vi "Create Instrument Addon From Configuration File.vi"(7 "Target in":refnum<k24>, 8 "error in (no error)":errorcluster, 11 "CD Config Path (.dat)":path) -> (0 "error out":errorcluster, 2 "Message Channels refnums":T2(array[cluster]) {"Message Group Ref" format="%.0x"; "Message Channels Refs" format="%.0x"}, 3 "Instrument Addon Refnum":T1=18446744073709551615 format="%.0x", 5 "Target out":refnum<k24>)   [LabVIEW 2018, in "Instrument Addon Scripting API.lvlib"]
uses:
  Instrument Addon Scripting API.lvlib
  <vilib>/NI Veristand/Custom Device API/Custom Device Item Ref.ctl
  NationalInstruments.VeriStand.SystemDefinitionAPI
  Addon/Addon Shared/SubVIs/Constants.vi
  <vilib>/NI Veristand/Custom Device Tools/Custom Device Utility Library/NI VeriStand - Search for All Items by GUID.vi
  <vilib>/NI Veristand/Custom Device Tools/Custom Device Utility Library/Custom Device Utility Library.lvlib
  Addon/Addon Shared/Instrument Addon Shared.lvlib
  <vilib>/NI/NI VeriStand Custom Device Import and Export Tool/ImportExport.lvlib
  <vilib>/NI Veristand/Custom Device API/Custom Device API.lvlib
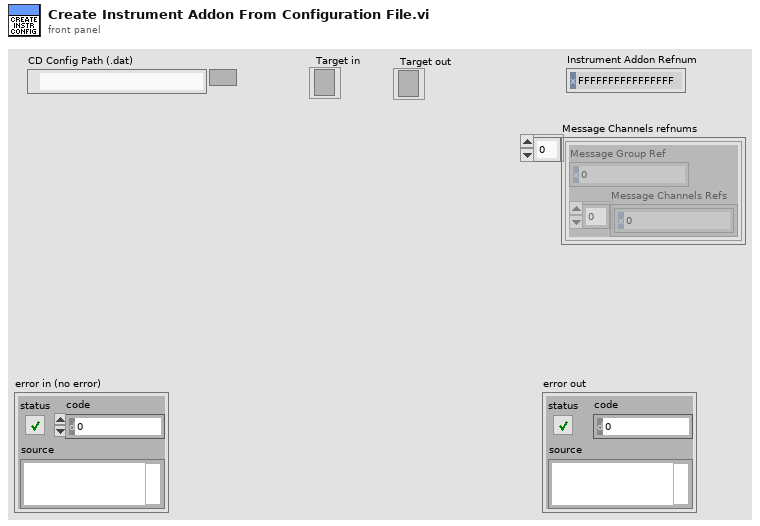
[diagram p1: front panel]
types:
  T1 = typedef "Custom Device API.lvlib/Custom Device Item Ref.ctl" = u64
  T2 = cluster{"Message Group Ref":T1, "Message Channels Refs":T1[]}[]
  T3 = cluster{"Message Group Ref":T1, "Message Channels Refs":T1[]}
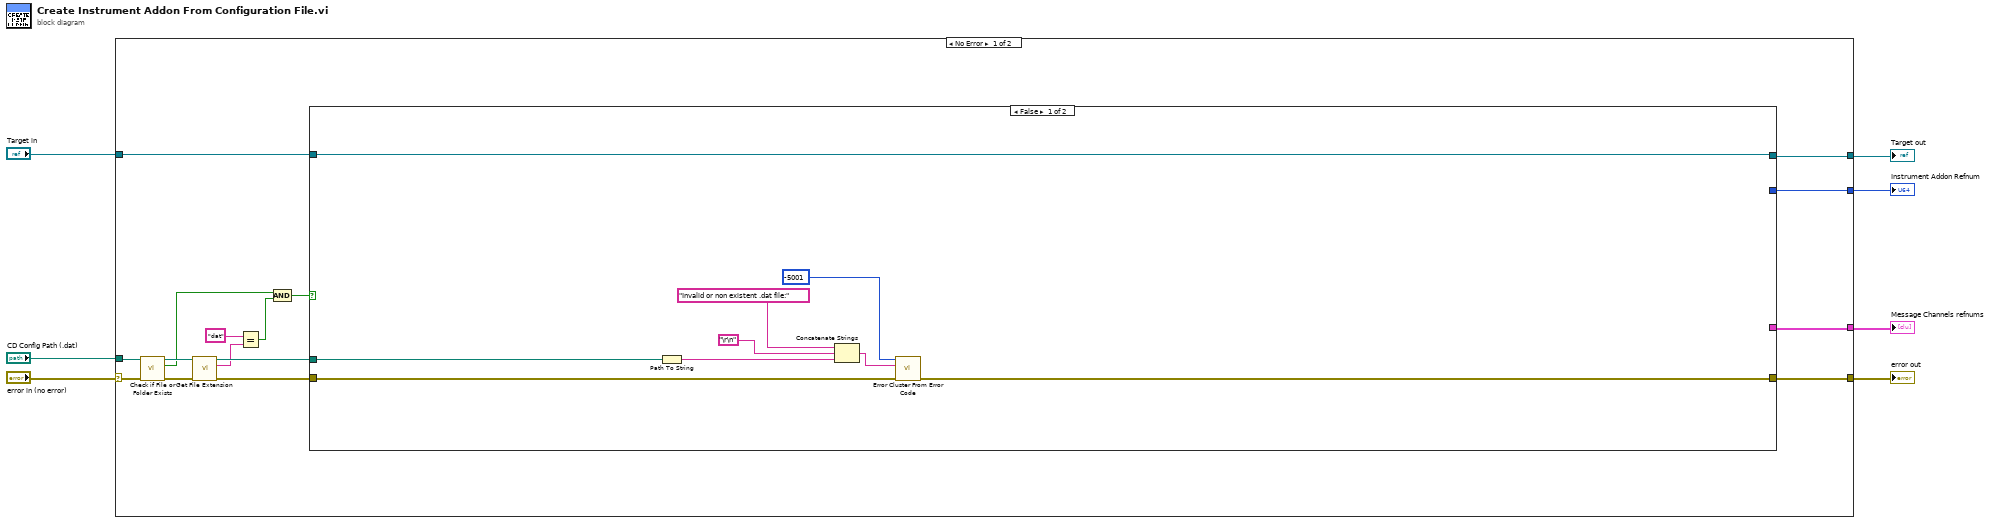
[diagram p0: block diagram]
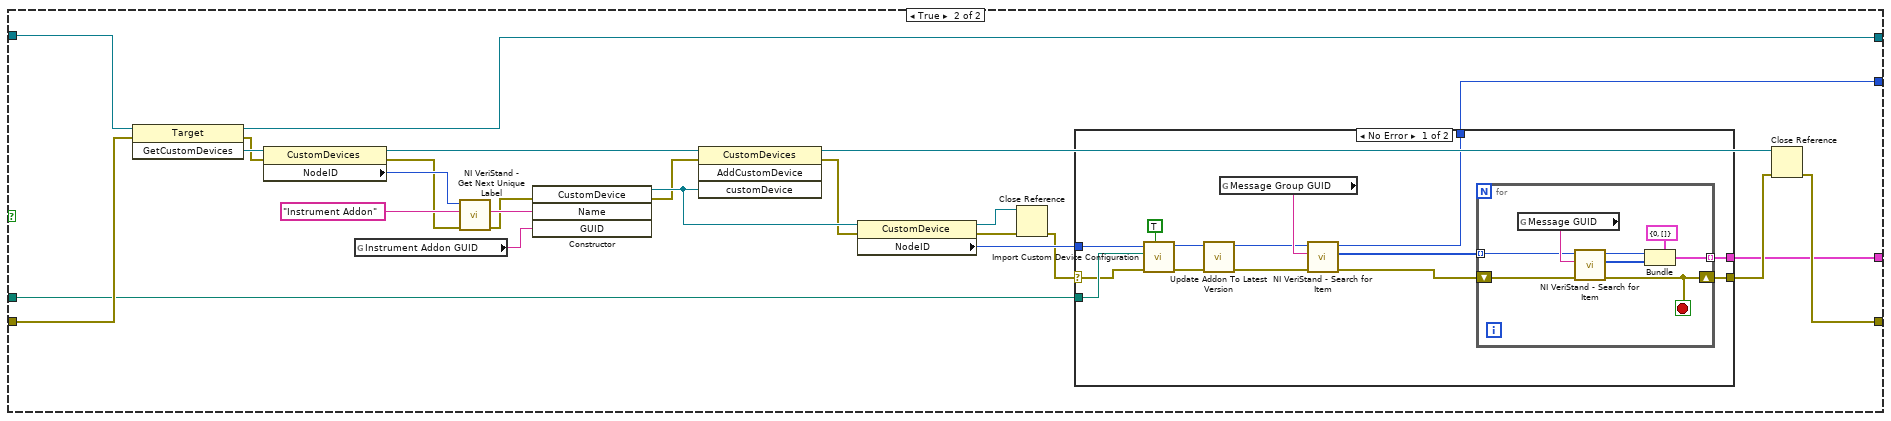
[diagram p2: hidden frame]
diagram:
  n1 = case shown="No Error" "error in (no error)" {
    selector: "error in (no error)" -> [w16 w83]
    tunnel: "Target in" -> [w23 w82]
    tunnel: [w22 w82] -> w6
    tunnel: "CD Config Path (.dat)" -> [w14 _]
    tunnel: [w21 w83] -> w4
    tunnel: [w20 _] -> w2
    tunnel: [w17 _] -> w1
    frame No Error {
      n2 = call <vilib>:"Check if File or Folder Exists.vi"("error in (no error)"=w16, "path"=w14) -> ("error out"=w15:errorcluster, "file or folder exists?"=w12:bool, "dup path"=w13:path)  [unwired: 7 in]
      n3 = call <vilib>:"Get File Extension.vi"("error in (no error)"=w15, "file"=w13) -> ("error out"=w19:errorcluster, "lowercase file extension"=w10:string, "dup file"=w18:path)  [unwired: 5 in, 2 out]
      n4 = Equal?(x="dat", y=w10) -> (x = y?=w8:bool)
      n5 = And(x=w12, y=w8) -> (x .and. y?=w11:bool)
      n6 = case shown="False" w11 {
        tunnel: w23 -> [w30 w56]
        tunnel: [w30 w55] -> w22
        tunnel: [w31 w54] -> w21
        tunnel: w19 -> [w32 w53]
        tunnel: [_ w44] -> w20
        tunnel: w18 -> [w28 w35]
        tunnel: [_ w34] -> w17
        frame False {
          n7 = Path To String(path=w28) -> (string=w27:string)
          n8 = Concatenate Strings("Invalid or non existent .dat file:" ("error message (\"\")"), "\r\n", w27) -> (w24:string)
          n9 = call <vilib>:"Error Cluster From Error Code.vi"("error in (no error)"=w32, "error message (\"\")"=w24, "error code (0)"=-5001) -> ("error out"=w31:errorcluster)  [unwired: 6 in]
        }
        frame True {
          n10 = invoke class="Target" method="GetCustomDevices"(reference=w56, error in=w53) -> (reference out=w55:refnum<k24>, error out=w42:errorcluster, "GetCustomDevices"=w43:refnum<k24>)  [unwired: 1 in]
          n11 = property class="CustomDevices"(reference=w43, error in=w42) -> (reference out=w39:refnum<k24>, error out=w37:errorcluster, "NodeID"=w41:u64)
          n12 = global read "Constants.vi" "Instrument Addon GUID"() -> (w46:string)
          n13 = call <vilib>:"NI VeriStand - Get Next Unique Label.vi"("error in (no error)"=w37, "Label"="Instrument Addon" ("Name"), "Parent Ref in"=w41) -> ("error out"=w36:errorcluster, "Label out"=w38:string)  [unwired: 5 in, 2 out]
          n14 = constructor class="CustomDevice"(error in=w36, "Name"=w38, "GUID"=w46) -> (reference out=w50:refnum<k24>, error out=w48:errorcluster)  [unwired: 2 in, 3 out]
          n15 = invoke class="CustomDevices" method="AddCustomDevice"(reference=w39, error in=w48, "customDevice"=w50) -> (reference out=w45:refnum<k24>, error out=w49:errorcluster)  [unwired: 1 in, 2 out]
          n16 = property class="CustomDevice"(reference=w50, error in=w49) -> (reference out=w51:refnum<k24>, error out=w52:errorcluster, "NodeID"=w47:u64)
          n17 = Close Reference(reference=w51, error in (no error)=w52) -> (error out=w33:errorcluster)
          n18 = case shown="No Error" w33 {
            selector: w33 -> [w58 w81]
            tunnel: [w69 w81] -> w57
            tunnel: w47 -> [w65 w80]
            tunnel: [w61 w80] -> w44
            tunnel: w35 -> [w60 _]
            tunnel: [w59 _] -> w34
            frame No Error {
              n19 = call <vilib>:"Import Custom Device Configuration.vi"("Overwrite Existing?"=TRUE, "error in (no error)"=w58, "Path"=w60, "NodeID"=w65) -> ("error out"=w67:errorcluster, "NodeID out"=w68:u64)  [unwired: 5 in, 1 out]
              n20 = call "Update Addon To Latest Version.vi"("error in (no error)"=w67, "Device Item Ref in"=w68) -> ("error out"=w63:errorcluster, "Device Item Ref out"=w64:T1)  [unwired: 8 in]
              n21 = global read "Constants.vi" "Message Group GUID"() -> (w71:string)
              n22 = call-poly <vilib>:"NI VeriStand - Search for Item.vi"("error in"=w63, "Item GUID"=w71, "Section Ref in"=w64) -> ("error out"=w62:errorcluster, "Item Refs"=w70:T1[], "Section Ref out"=w61:T1)  [unwired: 5 in, 1 out]
              n23 = for {
                tunnel: w70 -> [w78] mode=indexing
                tunnel: [w73] -> w59 mode=indexing
                shift-right: [w72] -> w69
                shift-left: w62 -> [w75]
                stop <- w72 stop-if-true
                n24 = global read "Constants.vi" "Message GUID"() -> (w79:string)
                n25 = call-poly <vilib>:"NI VeriStand - Search for Item.vi"("error in"=w75, "Item GUID"=w79, "Section Ref in"=w78) -> ("error out"=w72:errorcluster, "Item Refs"=w77:T1[], "Section Ref out"=w76:T1)  [unwired: 5 in, 1 out]
                n26 = Bundle(cluster=T3 {"Message Group Ref"=0, "Message Channels Refs"=[]}, "Message Group Ref"=w76, "Message Channels Refs"=w77) -> (w73:T3)
              }
            }
            frame Error {
            }
          }
          n27 = Close Reference(reference=w45, error in (no error)=w57) -> (error out=w54:errorcluster)
        }
      }
    }
    frame Error {
    }
  }
  "Message Channels refnums" <- w1
  "Target out" <- w6
  "error out" <- w4
  "Instrument Addon Refnum" <- w2
